vi "test case structure terminal detect.vi"() -> ()   [LabVIEW 2020, in "Method Generation.lvlib" / "Getter Generator.lvclass"]
uses:
  Getter Generator.lvclass
  <vilib>/Utility/traverseref.llb/TRef TravTarget.ctl
  Getter Generator.lvclass/Getter Generator.ctl
  test dummy.vi
  <vilib>/Utility/traverseref.llb/VI Scripting - Traverse.lvlib
panel:
  out "Method Generation.lvlib:Getter Generator.lvclass 2":refnum<class "Getter Generator.lvclass">
  in  "Method Generation.lvlib:Getter Generator.lvclass":refnum<class "Getter Generator.lvclass">
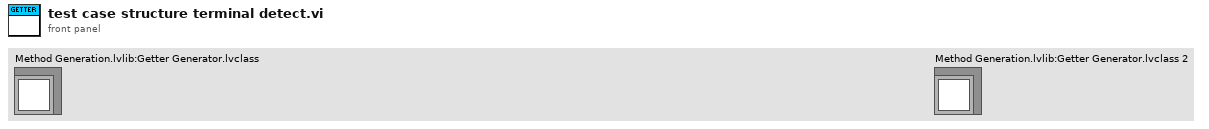
[diagram p1: front panel]
types:
  T1 = typedef "TRef TravTarget.ctl" = enum16{"FP", "BD", "Other"}
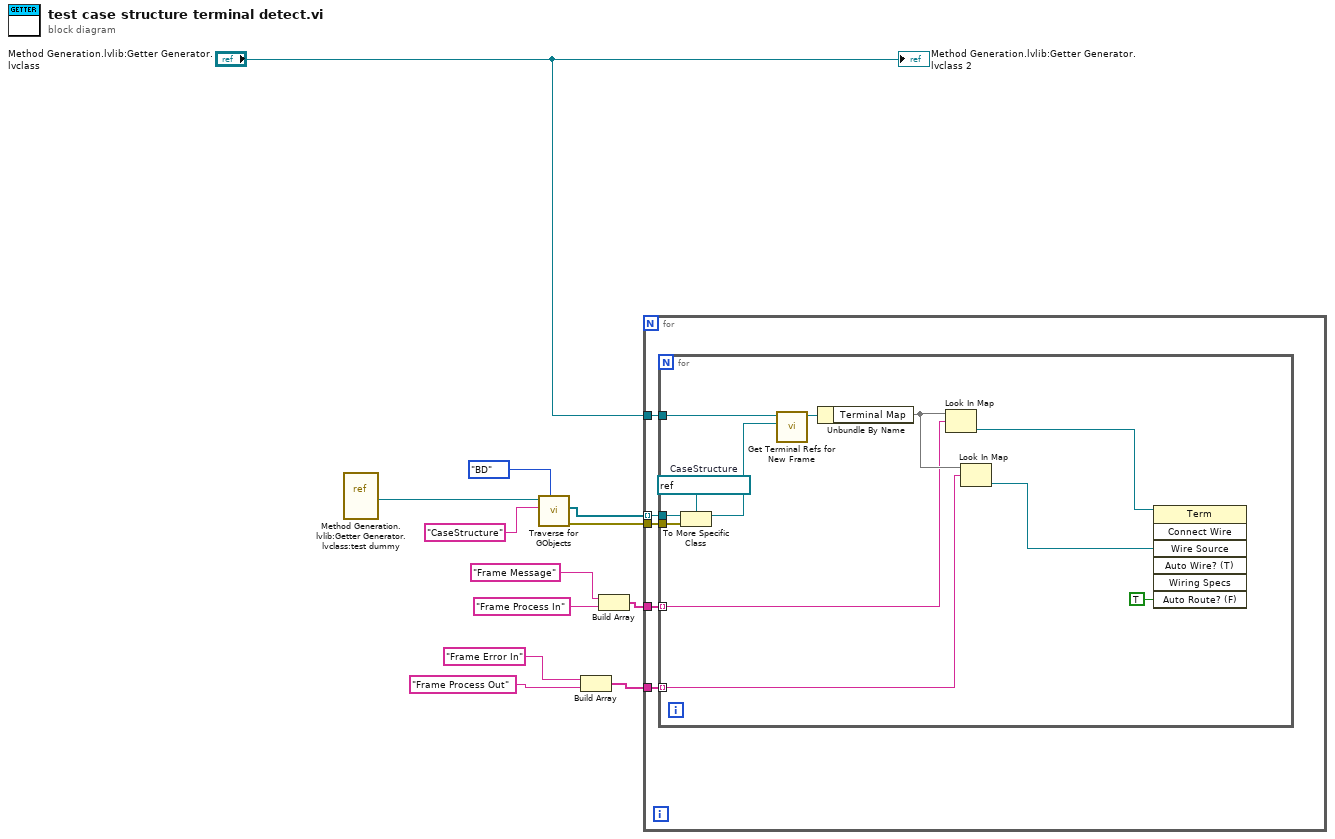
[diagram p0: block diagram]
diagram:
  n1 = vi-ref "Method Generation.lvlib:Getter Generator.lvclass:test dummy.vi"() -> (w7:refnum<vi>)
  n2 = call <vilib>:"Traverse for GObjects.vi"("Traverse Target"=TRef_TravTarget."BD", "Class Name"="CaseStructure", "VI Refnum"=w7) -> ("error out"=w9:errorcluster, "References"=w10:refnum<vi>[])  [unwired: 5 in, 2 out]
  n3 = Build Array("Frame Error In", "Frame Process Out") -> (w3:string[])
  n4 = Build Array("Frame Message", "Frame Process In") -> (w4:string[])
  n5 = for {
    tunnel: w10 -> [w17] mode=indexing
    tunnel: w9 -> [w16]
    tunnel: "Method Generation.lvlib:Getter Generator.lvclass" -> [w15]
    tunnel: w4 -> [w14]
    tunnel: w3 -> [w13]
    n6 = for {
      tunnel: w17 -> [w28]
      tunnel: w16 -> [w27]
      tunnel: w15 -> [w25]
      tunnel: w13 -> [w20] mode=indexing
      tunnel: w14 -> [w19] mode=indexing
      w29 = refnum<vi> refnum  # CaseStructure
      n7 = To More Specific Class(target class=w29, reference=w28, error in=w27) -> (specific class reference=w26:refnum<vi>)  [unwired: 1 out]
      n8 = call "Get Terminal Refs for New Frame.vi"("Case Structure Ref"=w26, "Getter Generator In"=w25) -> ("Getter Generator Out"=w24:refnum<class "Getter Generator.lvclass">)  [unwired: 7 in, 2 out]
      n9 = Unbundle By Name(w24) -> ("Terminal Map"=w23:map{string, refnum<vi>})
      n10 = Look In Map(map=w23, key=w19) -> (value=w22:refnum<vi>)  [unwired: 1 in, 1 out]
      n11 = Look In Map(map=w23, key=w20) -> (value=w21:refnum<vi>)  [unwired: 1 in, 1 out]
      n12 = invoke class="Term" method="Connect Wire"(reference=w22, "Wire Source"=w21, "Auto Route? (F)"=TRUE) -> ()  [unwired: 4 in, 7 out]
    }
  }
  "Method Generation.lvlib:Getter Generator.lvclass 2" <- "Method Generation.lvlib:Getter Generator.lvclass"
